vi "Write Partial.vi"(10 "Partial":bool, 11 "Series in":refnum<class "Series.lvclass">) -> (3 "Series out":refnum<class "Series.lvclass">)   [LabVIEW 2018, in "InfluxDB Client.lvlib" / "Series.lvclass"]
uses:
  Series.lvclass
  Series.lvclass/Series.ctl
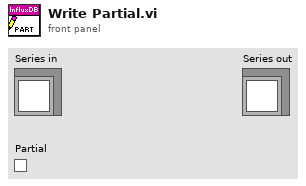
[diagram p1: front panel]
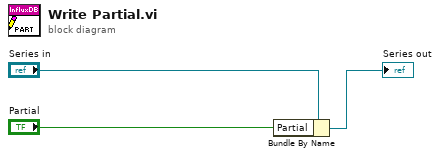
[diagram p0: block diagram]
diagram:
  n1 = Bundle By Name(cluster="Series in", "Partial"="Partial") -> (→"Series out":refnum<class "Series.lvclass">)
